vi "trig.vi"(8 "error in (no error)":errorcluster, 11 "5785_3.2GHz_one channel in":refnum<class "5785_3.2GHz_one channel.lvclass">) -> (0 "error out":errorcluster, 3 "5785_3.2GHz_one channel out":refnum<class "5785_3.2GHz_one channel.lvclass">)   [LabVIEW 2021, in "5785_3.2GHz_one channel.lvclass"]
uses:
  5785_3.2GHz_one channel.lvclass
  5785_3.2GHz_one channel.lvclass/5785_3.2GHz_one channel.ctl
  <instrlib>/_niInstr/Streaming/v1/Host/niInstr Streaming v1 Host.lvlib
  <instrlib>/_niInstr/Streaming/v1/Host/Public/Start Continuous Stream.vi
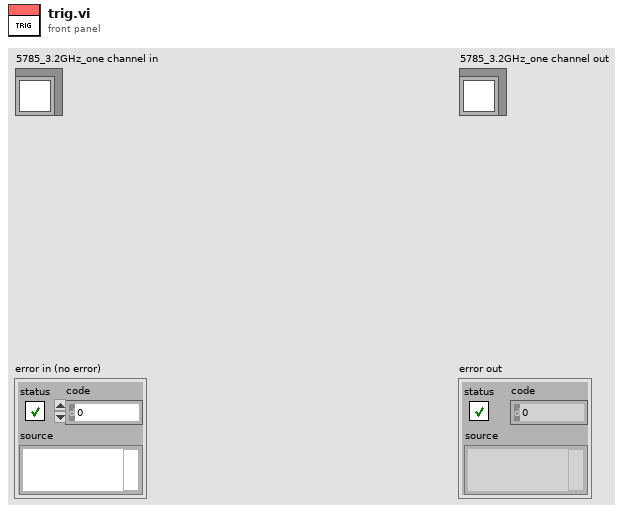
[diagram p1: front panel]
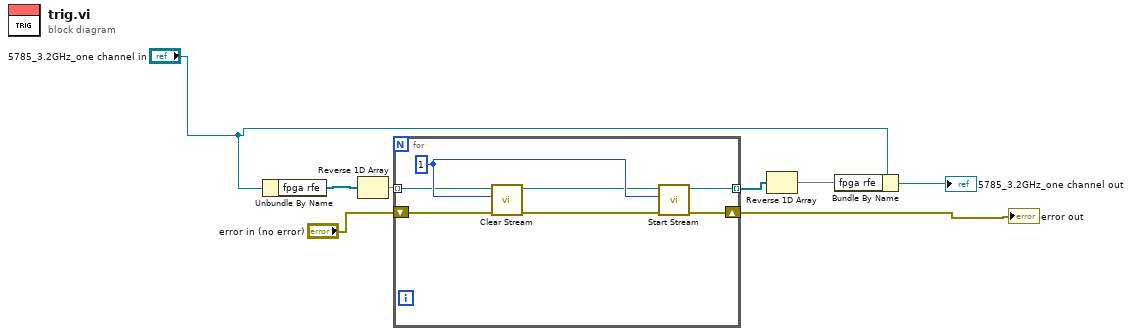
[diagram p0: block diagram]
diagram:
  n1 = Unbundle By Name("5785_3.2GHz_one channel in") -> ("fpga rfe"=w7:refnum<k20>[])
  n2 = Reverse 1D Array(array=w7) -> (reversed array=w8:refnum<k20>[])
  n3 = for {
    tunnel: w8 -> [w12] mode=indexing
    shift-right: [w14] -> w2
    shift-left: "error in (no error)" -> [w11]
    tunnel: [w13] -> w6 mode=indexing
    w15 = 1 ("stream index")
    n4 = call <instrlib>:"Clear Stream.vi"("error in (no error)"=w11, "stream index"=w15, "refnum in"=w12) -> ("error out"=w10:errorcluster, "refnum out"=w9:refnum<k20>)  [unwired: 7 in]
    n5 = call-poly <instrlib>:"Start Stream.vi"("error in (no error)"=w10, "stream index"=w15, "refnum in"=w9) -> ("error out"=w14:errorcluster, "refnum out"=w13:refnum<k20>)  [unwired: 7 in]
  }
  "error out" <- w2
  n6 = Reverse 1D Array(array=w6) -> (reversed array=w5:refnum<k20>[])
  n7 = Bundle By Name(cluster="5785_3.2GHz_one channel in", "fpga rfe"=w5) -> (→"5785_3.2GHz_one channel out":refnum<class "5785_3.2GHz_one channel.lvclass">)
